vi "Stop Core.vi"(10 "final error code":i32, 11 "Generic Instrument in":refnum<class "Generic Instrument.lvclass">) -> (3 "Generic Instrument out":refnum<class "Generic Instrument.lvclass">)   [LabVIEW 2014, in "Generic Instrument.lvlib" / "Generic Instrument.lvclass"]
doc: "(<B>Filename</B>: Actor Framework.lvlib:Actor.lvclass:Stop Core.vi)\n\nDefines what the actor does before it stops. Use the <B>final error code</B> input to determine whether the actor shut down in response to an error.\n\nBy default, this method does nothing. A descendant class may override it to define behavior, such as shutting down any processes the actor initiated in its override of the Actor Core method."
uses:
  Generic Instrument.lvclass
  Subpanel Insertion/Subpanel Inserter.lvclass
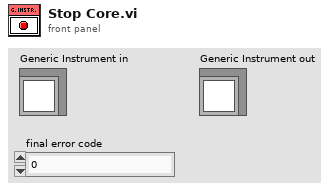
[diagram p1: front panel]
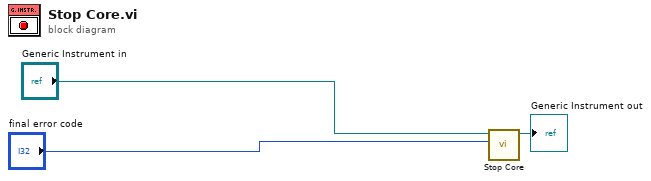
[diagram p0: block diagram]
diagram:
  n1 = call-parent "Stop Core.vi"("final error code"="final error code", "Subpanel Inserter in"="Generic Instrument in") -> ("Subpanel Inserter out"=→"Generic Instrument out":refnum<class "Generic Instrument.lvclass">)  [unwired: 9 in]
